vi "Write name.vi"(5 "name":string, 9 "Node in":refnum<class "Node.lvclass">) -> (3 "Node out":refnum<class "Node.lvclass">)   [LabVIEW 2014, in "Raspberry Pi Compatible Compiler for LabVIEW.lvlib" / "Node.lvclass"]
uses:
  Node.lvclass
  Node.lvclass/Node.ctl
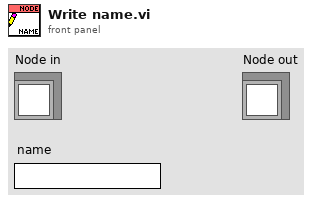
[diagram p1: front panel]
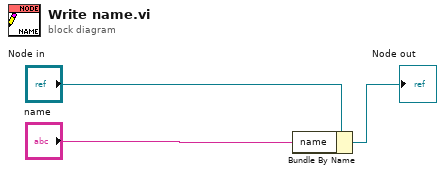
[diagram p0: block diagram]
diagram:
  n1 = Bundle By Name(cluster="Node in", "name"="name") -> (→"Node out":refnum<class "Node.lvclass">)
